vi "SpinnyGloDebugger.vi"() -> ()   [LabVIEW 2014]
uses:
  <vilib>/userdefined/High Color/IMAQdx.ctl
  <vilib>/LabVIEW Interface for Arduino/LabVIEW Interface for Arduino.lvlib
  <vilib>/vision/driver/NI_Vision_Acquisition_Software.lvlib
panel:
  in  "Camera 2 Name":T1
  out "Image 2":T2(plugin-control)
  out "Steps per Image":dbl
  out "Total Steps":dbl
  out "Images Acquired":i32
  in  "File Name":string
  in  "Save Location":path
  out "Image":T2(plugin-control)
  out "Degrees per Step":dbl
  out "Degrees per Image":dbl
  in  "Number of Images":dbl
  in  "Camera 1 Name":T1
  out "Steps Remaining":u32
  in  "Angular Increment":dbl
  in  "Exit":bool
  in  "Home":bool
  in  "Stop":bool
  in  "MoveToGo":bool
  in  "MoveForGo":bool
  in  "Direction":bool
  out "Current Position":dbl format="%#.2f"
  in  "Move For (+/-360 max)":dbl
  in  "Move To":dbl
  # "CW"
  # "CCW"
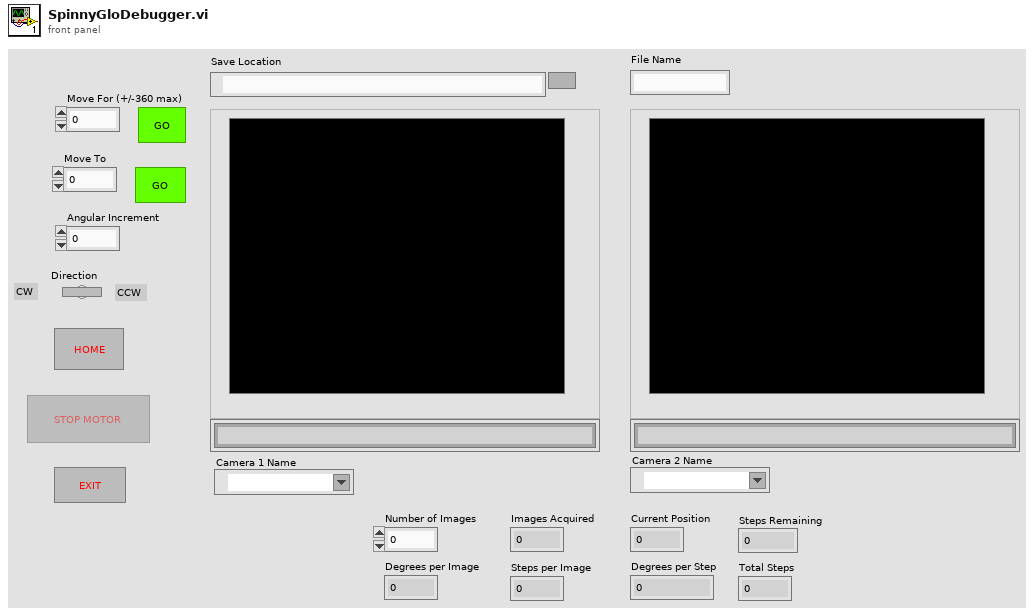
[diagram p1: front panel]
types:
  T1 = typedef "IMAQdx.ctl" = refnum<k21>
  T2 = typedef "IMAQ Image.ctl" = refnum<image>
  T3 = enum16{"Enabled", "Disabled", "Disabled and Grayed Out"}
  T4 = enum8{"Enabled", "Disabled", "Disabled and Grayed Out"}
  T5 = typedef "LabVIEW Interface for Arduino.lvlib/Arduino Resource.ctl" = cluster{"VISA resource":refnum<visa-resource-name>, "Board Type":T6, "Connection Type":enum8{"USB / Serial"}, "Bytes Per Packet (15)":u8}
  T6 = typedef "LabVIEW Interface for Arduino.lvlib/Board Type.ctl" = enum16{"Uno", "Dimuelanove w/Atmega 328", "Mega 2560"}
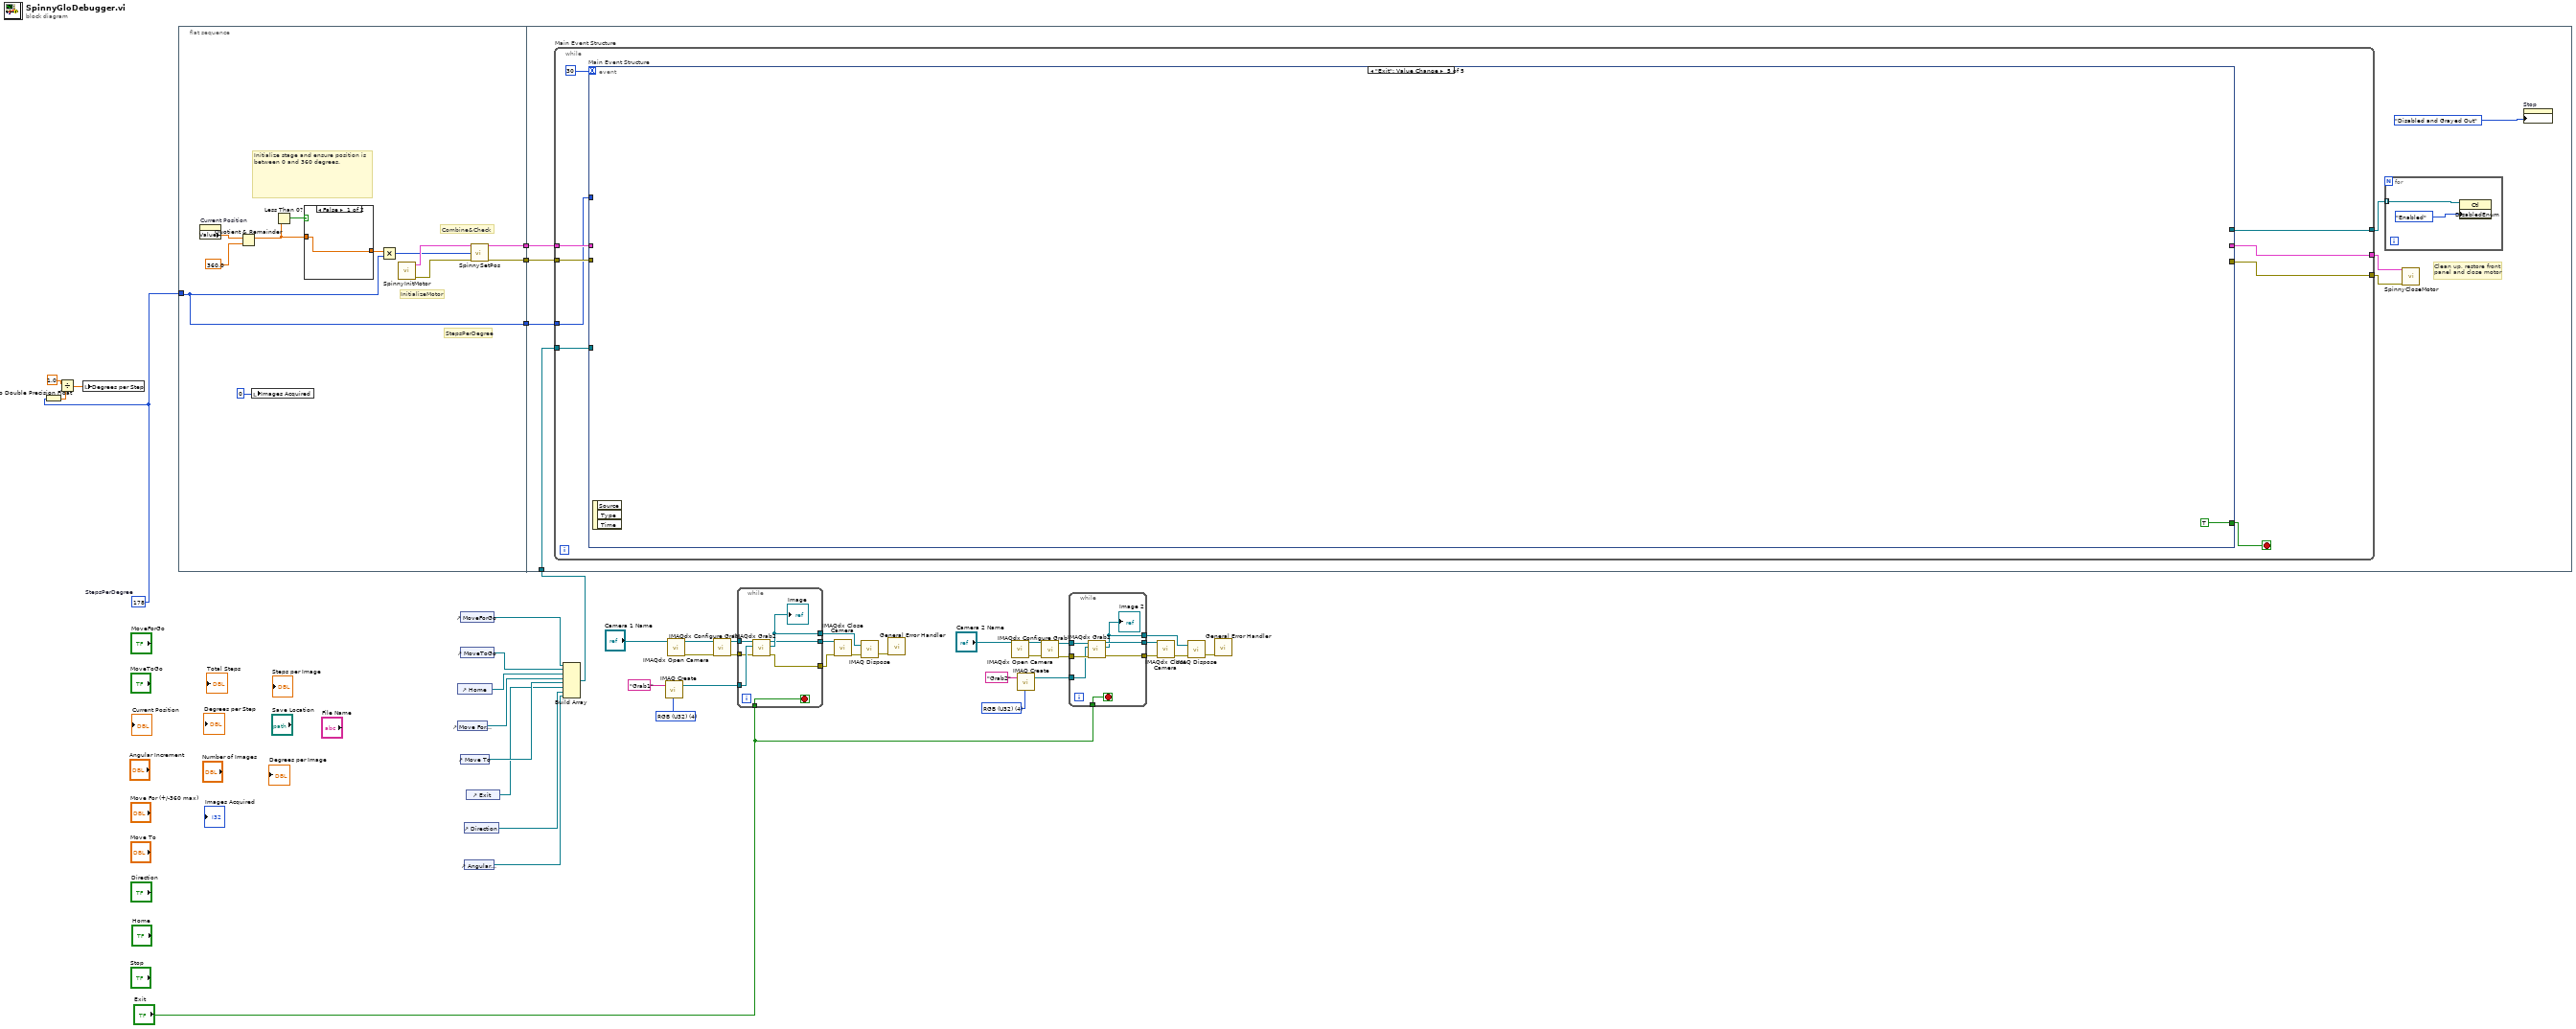
[diagram p0: block diagram]
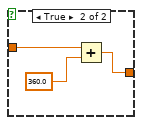
[diagram p2: hidden frame]
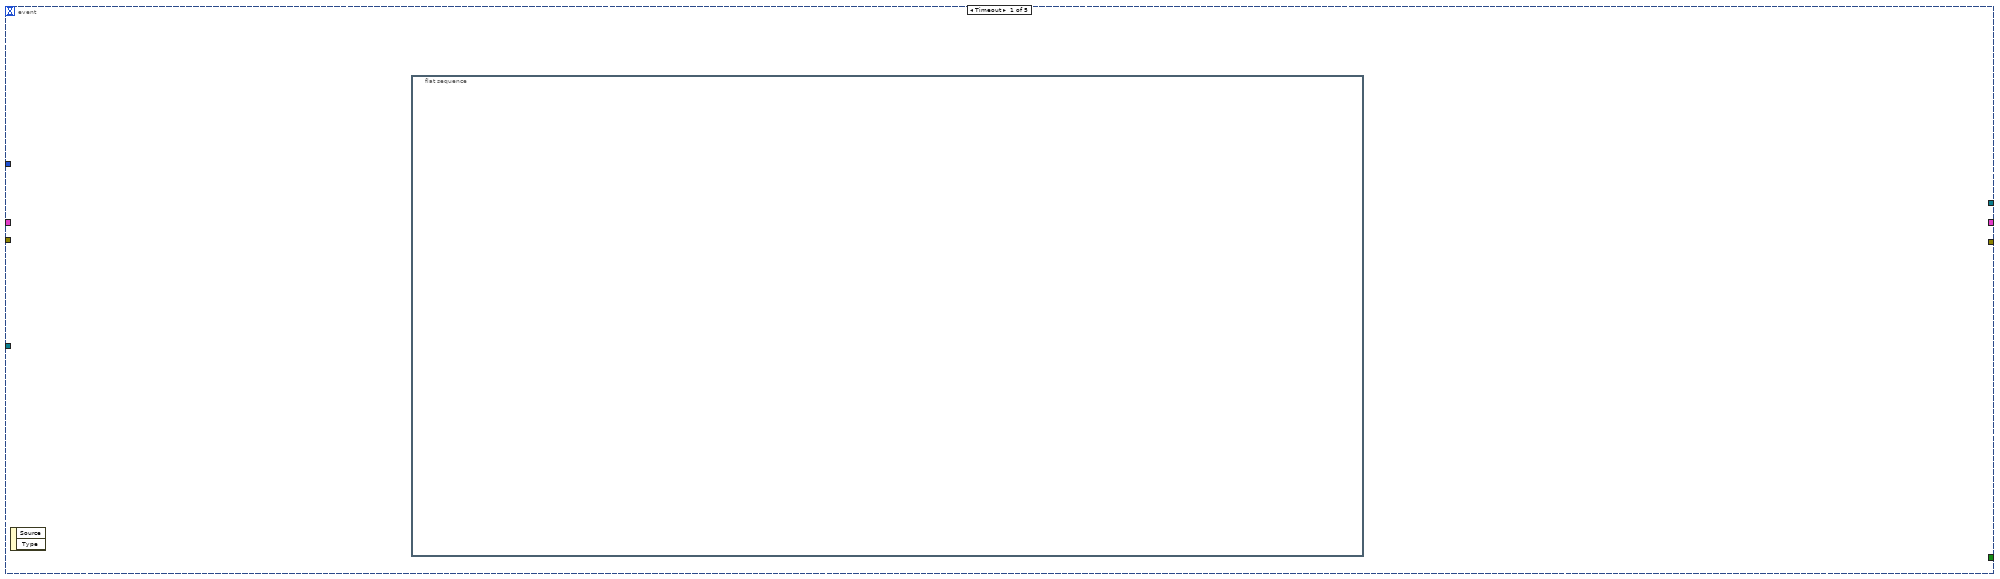
[diagram p3: hidden frame]
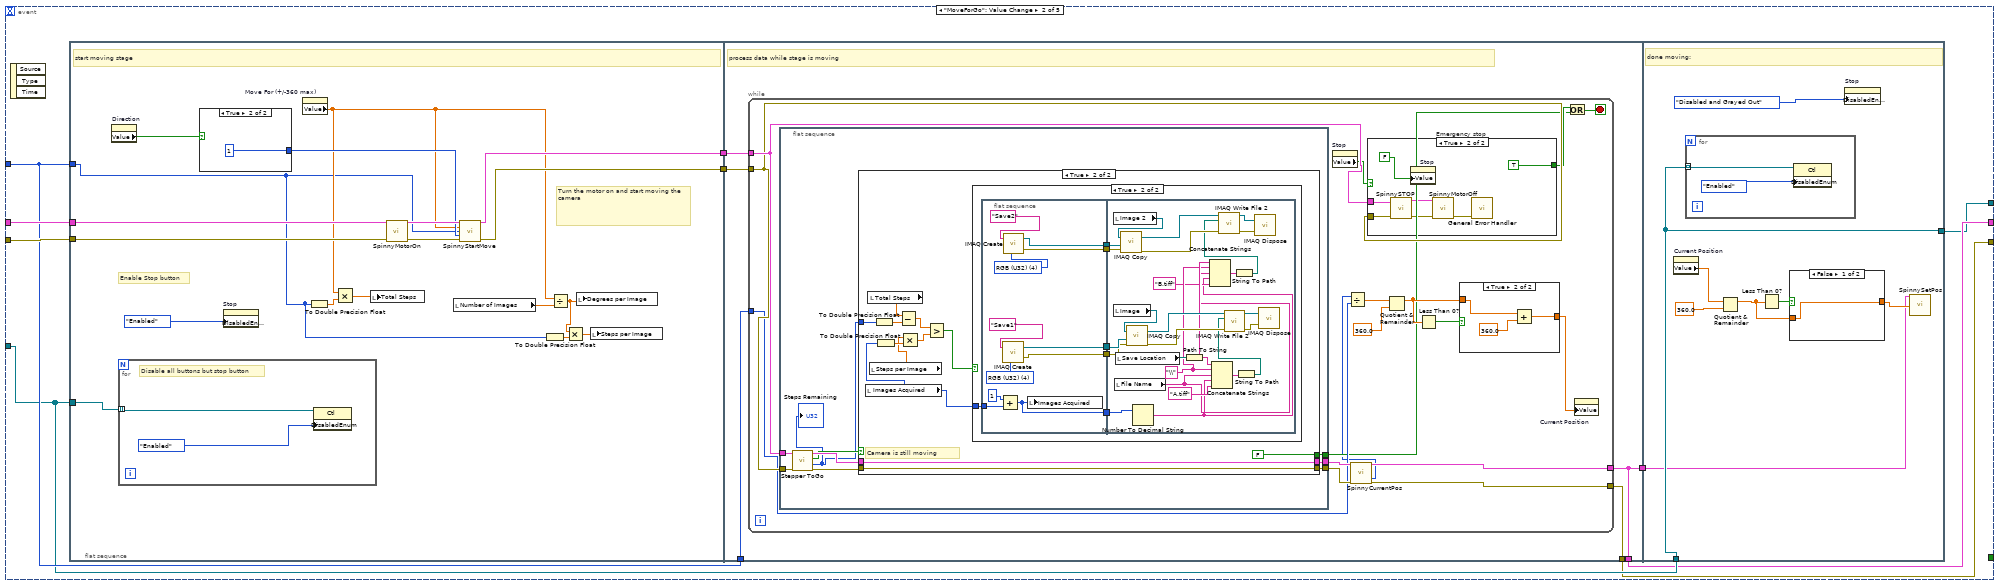
[diagram p4: hidden frame]
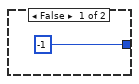
[diagram p5: hidden frame]
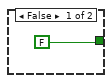
[diagram p7: hidden frame]
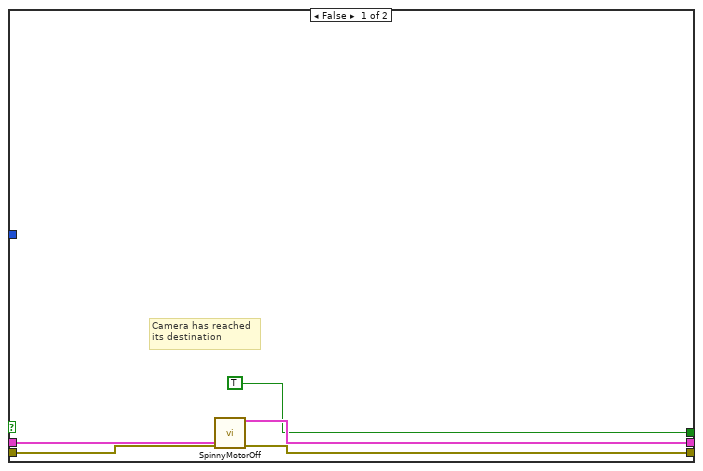
[diagram p8: hidden frame]
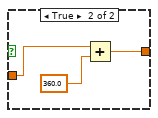
[diagram p10: hidden frame]
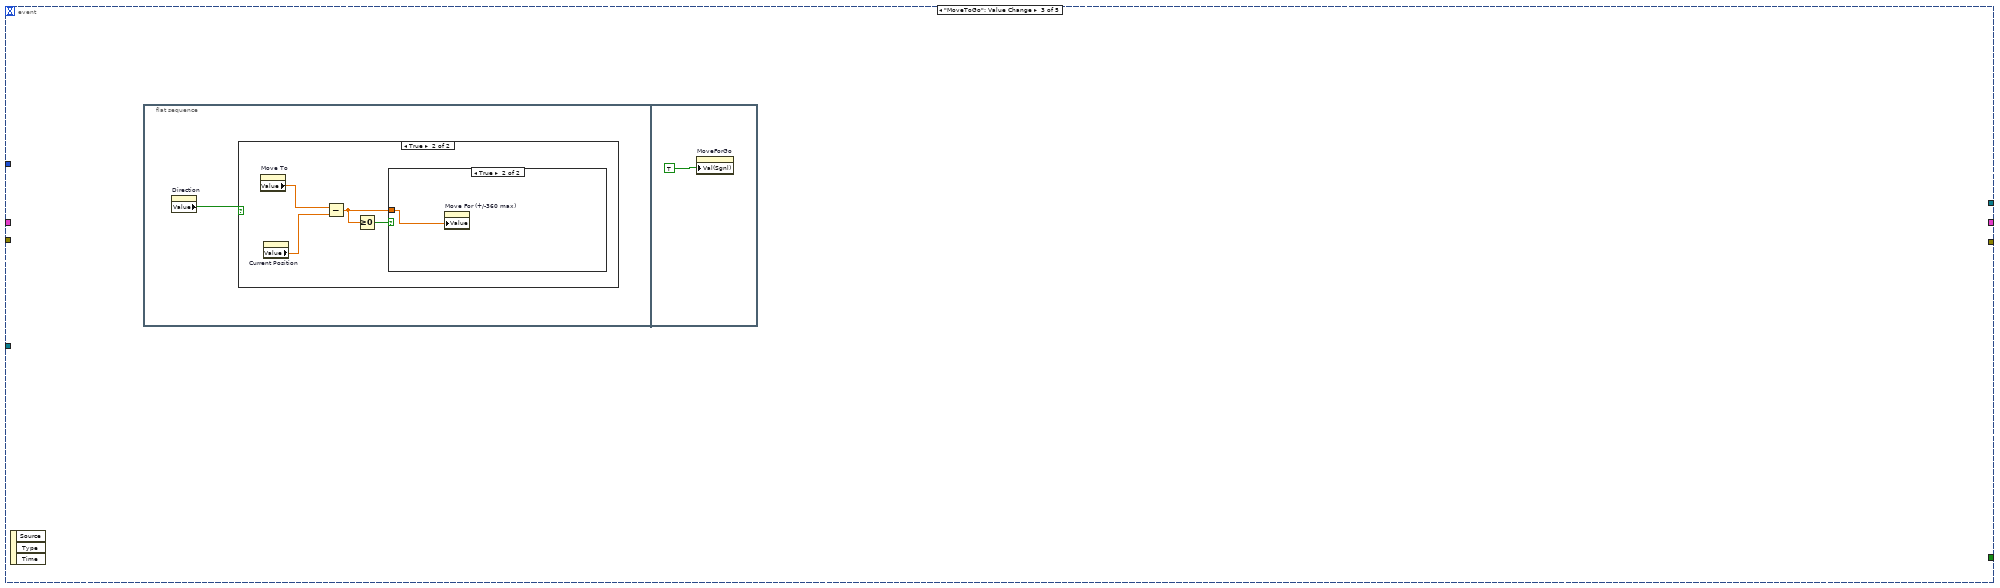
[diagram p11: hidden frame]
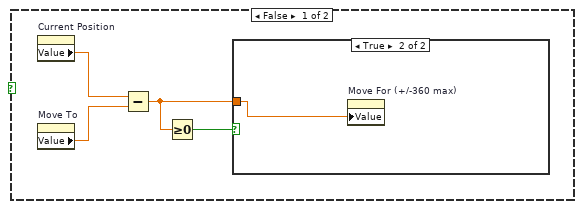
[diagram p12: hidden frame]
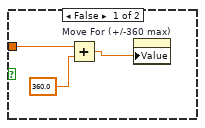
[diagram p13: hidden frame]
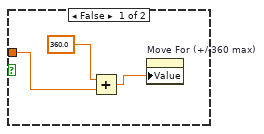
[diagram p14: hidden frame]
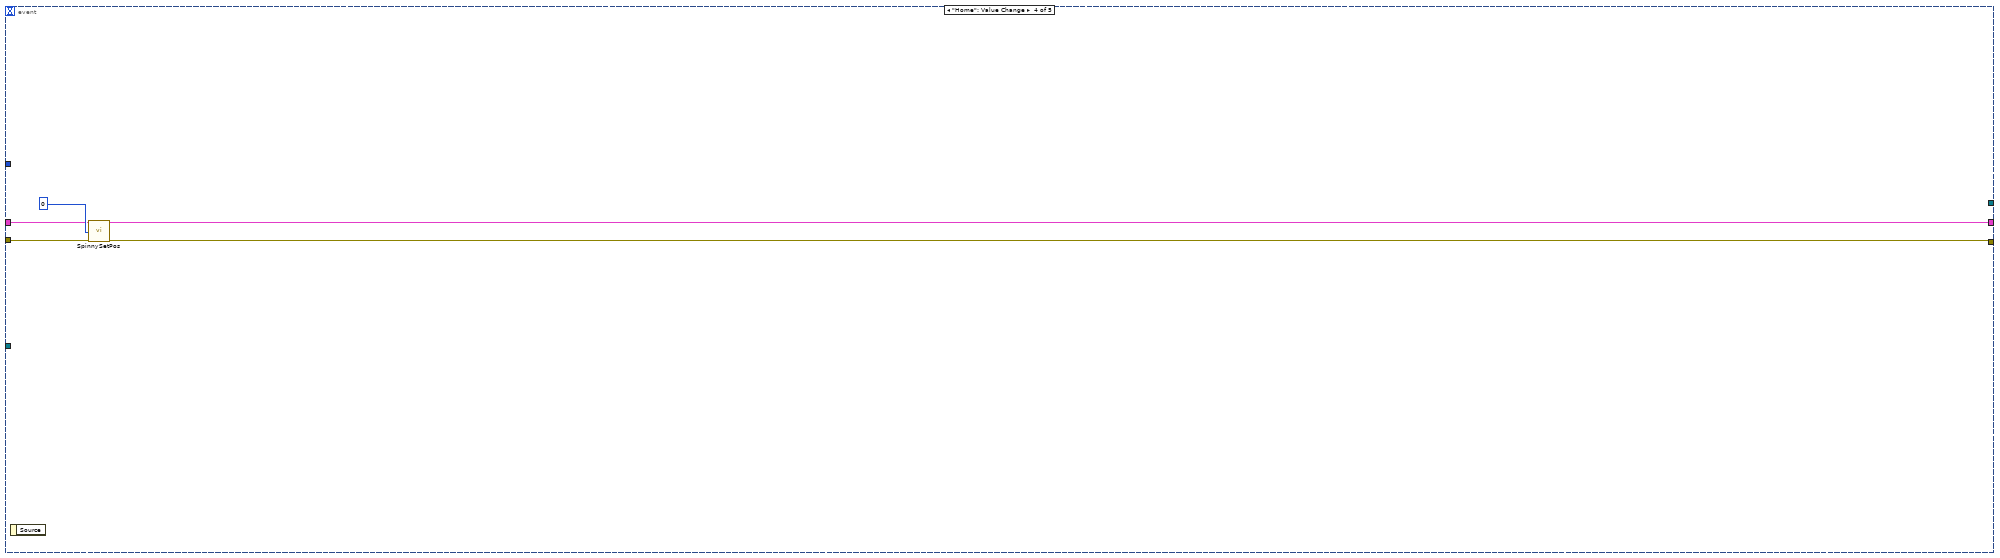
[diagram p15: hidden frame]
diagram:
  w11 = u32 4 items=["Grayscale (U8)", "Grayscale (I16)", "Grayscale (SGL)", "Complex (CSG)", "RGB (U32)", "HSL (U32)", "RGB (U64)", "Grayscale (U16)", ""] ("Image Type")
  w31 = u32 4 items=["Grayscale (U8)", "Grayscale (I16)", "Grayscale (SGL)", "Complex (CSG)", "RGB (U32)", "HSL (U32)", "RGB (U64)", "Grayscale (U16)", ""] ("Image Type")
  w15 = 178  # StepsPerDegree
  n1 = To Double Precision Float(number=w15) -> (double precision float=w18:dbl)
  n2 = Divide(x=1.0, y=w18) -> (x/y=w16:dbl)
  n3 = local write "Degrees per Step"(w16) -> ()
  n4 = flat-sequence {
    tunnel: w15 -> [w45]
    tunnel: [w47] -> w43
    tunnel: [w46] -> w42
    tunnel: [w45] -> w32
    tunnel: w43 -> [w66]
    tunnel: w42 -> [w65]
    tunnel: w33 -> [w67]
    tunnel: w32 -> [w64]
    frame #0 {
      # "StepsPerDegree"
      # "Combine&Check"
      # "InitializeMotor"
      # "Initialize stage and ensure position is between 0 and 360 degrees."
      n5 = property on="Current Position" class="DigNum (strict)"() -> ("Value"=w55:dbl)  [unwired: 2 in, 2 out]
      n6 = Quotient & Remainder(x=w55, y=sgl 360.0) -> (x-y*floor(x/y)=w52:dbl)  [unwired: 1 out]
      n7 = local write "Images Acquired"(0) -> ()
      n8 = Less Than 0?(x=w52) -> (x < 0?=w53:bool)
      n9 = case shown="False" w53 {
        tunnel: w52 -> [w56 w59]
        tunnel: [w56 w57] -> w51
        frame False {
        }
        frame True {
          n10 = Add(x=w59, y=sgl 360.0) -> (x+y=w57:dbl)
        }
      }
      n11 = Multiply(x=w51, y=w45) -> (x*y=w48:i32)
      n12 = call "SpinnyInitMotor.vi"() -> ("error out"=w49:errorcluster, "Arduino Resource Out"=w50:T5)  [unwired: 10 in]
      n13 = call "SpinnySetPos.vi"("Arduino Resource"=w50, "position"=w48, "error in"=w49) -> ("Arduino Resource Out"=w47:T5, "error out"=w46:errorcluster)  [unwired: 15 in]
    }
    frame #1 {
      # "Clean up, restore front\npanel and close motor"
      n14 = while "Main Event Structure" {
        tunnel: w67 -> [w77]
        tunnel: w66 -> [w76]
        tunnel: w65 -> [w75]
        tunnel: w64 -> [w74]
        tunnel: [w73] -> w61
        tunnel: [w72] -> w63
        tunnel: [w71] -> w62
        stop <- w70 stop-if-true
        n15 = event "Main Event Structure" shown="[4] \"Exit\": Value Change" {
          selector: _ -> [_ _ _ _ _]
          dyn-events: _ -> [_ _ _ _ _]
          timeout: 30 -> [_ _ _ _ _]
          tunnel: w77 -> [_ w82 _ _ _]
          tunnel: w76 -> [_ w88 _ w249 _]
          tunnel: w75 -> [_ w87 _ w248 _]
          tunnel: w74 -> [_ w84 _ _ _]
          tunnel: [_ w81 _ w247 _] -> w72
          tunnel: [_ w80 _ w246 _] -> w71
          tunnel: [_ w79 _ _ _] -> w73
          tunnel: [_ _ _ _ TRUE] -> w70
          event Timeout {
            n16 = event-data() -> ()  [unwired: 1 in, 2 out]
            n17 = flat-sequence {
              frame #0 {
              }
            }
          }
          event "MoveForGo": Value Change {
            n18 = event-data() -> ()  [unwired: 1 in, 3 out]
            n19 = flat-sequence {
              tunnel: w82 -> [w106]
              tunnel: w88 -> [w103]
              tunnel: w87 -> [w101]
              tunnel: w84 -> [w92]
              tunnel: [w98] -> w86
              tunnel: [w97] -> w85
              tunnel: w86 -> [w115]
              tunnel: w85 -> [w114]
              tunnel: w84 -> [w113]
              tunnel: [w112] -> w83
              tunnel: [w112] -> w81
              tunnel: [w111] -> w80
              tunnel: w83 -> [w214]
              tunnel: w82 -> [w215]
              tunnel: [w215] -> w79
              frame #0 {
                # "Turn the motor on and start moving the camera"
                # "start moving stage"
                # "Enable Stop button"
                n20 = property on="Direction" class="Bool (strict)"() -> ("Value"=w104:bool)  [unwired: 2 in, 2 out]
                n21 = for {
                  tunnel: w106 -> [w110] mode=indexing
                  # "Disable all buttons but stop button"
                  n22 = property class="Ctl"(reference=w110, "DisabledEnum"=T3."Enabled") -> ()  [unwired: 1 in, 2 out]
                }
                n23 = case shown="True" w104 {
                  tunnel: [-1 1] -> w99
                  frame False {
                  }
                  frame True {
                  }
                }
                n24 = property on="Stop" class="Bool (strict)"("DisabledEnum"=T4."Enabled") -> ()  [unwired: 2 in, 2 out]
                n25 = property on="Move For (+/-360 max)" class="DigNum (strict)"() -> ("Value"=w94:dbl)  [unwired: 2 in, 2 out]
                n26 = To Double Precision Float(number=w92) -> (double precision float=w95:dbl)
                n27 = Multiply(x=w94, y=w95) -> (x*y=w93:dbl)
                n28 = local write "Total Steps"(w93) -> ()
                n29 = call "SpinnyMotorOn.vi"("Arduino Resource"=w103, "error in"=w101) -> ("Arduino Resource Out"=w102:T5, "error out"=w100:errorcluster)  [unwired: 12 in]
                n30 = local read "Number of Images"() -> (w96:dbl)
                n31 = call "SpinnyStartMove.vi"("Arduino Resource"=w102, "Degrees To Move"=w94, "Steps Per Degree"=w92, "Direction"=w99, "error in"=w100) -> ("Arduino Resource Out"=w98:T5, "error out"=w97:errorcluster)  [unwired: 9 in]
                n32 = To Double Precision Float(number=w92) -> (double precision float=w91:dbl)
                n33 = Divide(x=w94, y=w96) -> (x/y=w90:dbl)
                n34 = Multiply(x=w90, y=w91) -> (x*y=w89:dbl)
                n35 = local write "Degrees per Image"(w90) -> ()
                n36 = local write "Steps per Image"(w89) -> ()
              }
              frame #1 {
                # "process data while stage is moving"
                n37 = while {
                  tunnel: w115 -> [w130]
                  tunnel: w114 -> [w129]
                  tunnel: [w128] -> w111
                  tunnel: [w126] -> w112
                  tunnel: w113 -> [w125]
                  stop <- w118 stop-if-true
                  n38 = flat-sequence {
                    tunnel: w129 -> [w153]
                    tunnel: w130 -> [w152]
                    tunnel: [w148] -> w131
                    tunnel: [w147] -> w132
                    tunnel: [w146] -> w119
                    frame #0 {
                      n39 = call <vilib>:"Stepper ToGo.vi"("error in"=w153, "Arduino Resource"=w152) -> ("error out"=w150:errorcluster, "Steps remaining"=w145:u32, "Steps Remaining?"=w149:bool, "Arduino Resource Out"=w151:T5)  [unwired: 6 in]
                      "Steps Remaining" <- w145
                      n40 = case shown="True" w149 {
                        tunnel: w151 -> [w158 w170]
                        tunnel: w150 -> [w157 w169]
                        tunnel: [w156 w170] -> w147
                        tunnel: [w155 w169] -> w148
                        tunnel: [TRUE FALSE] -> w146
                        tunnel: w145 -> [_ w167]
                        frame False {
                          # "Camera has reached\nits destination"
                          n41 = call "SpinnyMotorOff.vi"("Arduino Resource"=w158, "error in"=w157) -> ("Arduino Resource Out"=w156:T5, "error out"=w155:errorcluster)  [unwired: 12 in]
                        }
                        frame True {
                          # "Camera is still moving"
                          n42 = local read "Images Acquired"() -> (w161:i32)
                          n43 = local read "Total Steps"() -> (w165:dbl)
                          n44 = local read "Steps per Image"() -> (w160:dbl)
                          n45 = To Double Precision Float(number=w167) -> (double precision float=w166:dbl)
                          n46 = To Double Precision Float(number=w161) -> (double precision float=w162:dbl)
                          n47 = Subtract(x=w165, y=w166) -> (x-y=w164:dbl)
                          n48 = Multiply(x=w160, y=w162) -> (x*y=w159:dbl)
                          n49 = Greater?(x=w164, y=w159) -> (0:w163:bool)
                          n50 = case shown="True" w163 {
                            tunnel: w161 -> [_ w174]
                            frame False {
                            }
                            frame True {
                              n51 = flat-sequence {
                                tunnel: [w185] -> w176
                                tunnel: [w184] -> w175
                                tunnel: w174 -> [w183]
                                tunnel: [w181] -> w173
                                tunnel: [w178] -> w172
                                tunnel: [w177] -> w171
                                tunnel: w176 -> [w212]
                                tunnel: w175 -> [w208]
                                tunnel: w173 -> [w204]
                                tunnel: w172 -> [w195]
                                tunnel: w171 -> [w194]
                                frame #0 {
                                w179 = u16 4 items=["Grayscale (U8)", "Grayscale (I16)", "Grayscale (SGL)", "Complex (CSG)", "RGB (U32)", "HSL (U32)", "RGB (U64)", "Grayscale (U16)", ""]
                                w186 = u16 4 items=["Grayscale (U8)", "Grayscale (I16)", "Grayscale (SGL)", "Complex (CSG)", "RGB (U32)", "HSL (U32)", "RGB (U64)", "Grayscale (U16)", ""]
                                n52 = Add(x=1, y=w183) -> (x+y=w181:i32)
                                n53 = call "IMAQ Create"("Image Name"="Save1", "Image Type"=w186) -> ("New Image"=w185:T2, "error out"=w184:errorcluster)  [unwired: 3 in]
                                n54 = call "IMAQ Create"("Image Name"="Save2", "Image Type"=w179) -> ("New Image"=w178:T2, "error out"=w177:errorcluster)  [unwired: 3 in]
                                n55 = local write "Images Acquired"(w181) -> ()
                                }
                                frame #1 {
                                w200 = "\\"
                                n56 = local read "Image 2"() -> (w196:T2)
                                n57 = local read "Image"() -> (w213:T2)
                                n58 = local read "File Name"() -> (w199:string)
                                n59 = local read "Save Location"() -> (w206:path)
                                n60 = call "IMAQ Copy"("error in (no error)"=w194, "Image Dst"=w195, "Image Src"=w196) -> ("error out"=w193:errorcluster, "Image Dst Out"=w191:T2)  [unwired: 3 in]
                                n61 = call "IMAQ Copy"("error in (no error)"=w208, "Image Dst"=w212, "Image Src"=w213) -> ("error out"=w207:errorcluster, "Image Dst Out"=w211:T2)  [unwired: 3 in]
                                n62 = Number To Decimal String(number=w204) -> (decimal integer string=w197:string)  [unwired: 1 in]
                                n63 = Path To String(path=w206) -> (string=w201:string)
                                n64 = Concatenate Strings(w201, w200, w199, w197, "B.tiff") -> (w189:string)
                                n65 = Concatenate Strings(w201, w200, w199, w197, "A.tiff") -> (w203:string)
                                n66 = String To Path(string=w189) -> (path=w188:path)
                                n67 = call-poly "IMAQ Write File 2"("error in (no error)"=w193, "File Path"=w188, "Image"=w191) -> ("error out"=w192:errorcluster, "Image Out (duplicate)"=w190:T2)  [unwired: 7 in]
                                n68 = String To Path(string=w203) -> (path=w202:path)
                                n69 = call-poly "IMAQ Write File 2"("error in (no error)"=w207, "File Path"=w202, "Image"=w211) -> ("error out"=w209:errorcluster, "Image Out (duplicate)"=w210:T2)  [unwired: 7 in]
                                n70 = call "IMAQ Dispose"("Image"=w190, "error in (no error)"=w192) -> ()  [unwired: 4 in, 1 out]
                                n71 = call "IMAQ Dispose"("Image"=w210, "error in (no error)"=w209) -> ()  [unwired: 4 in, 1 out]
                                }
                              }
                            }
                          }
                        }
                      }
                    }
                  }
                  n72 = property on="Stop" class="Bool (strict)"() -> ("Value"=w127:bool)  [unwired: 2 in, 2 out]
                  n73 = call "SpinnyCurrentPos.vi"("Arduino Resource"=w132, "error in"=w131) -> ("Arduino Resource Out"=w126:T5, "position"=w116:i32, "error out"=w128:errorcluster)  [unwired: 15 in]
                  n74 = Divide(x=w116, y=w125) -> (x/y=w124:dbl)
                  n75 = case "Emergency stop" shown="True" w127 {
                    tunnel: w130 -> [_ w144]
                    tunnel: w129 -> [_ w142]
                    tunnel: [FALSE TRUE] -> w120
                    frame False {
                    }
                    frame True {
                      n76 = call "SpinnySTOP.vi"("error in"=w142, "Arduino Resource"=w144) -> ("error out"=w141:errorcluster, "Arduino Resource Out"=w143:T5)  [unwired: 8 in]
                      n77 = property on="Stop" class="Bool (strict)"("Value"=FALSE) -> ()  [unwired: 2 in, 2 out]
                      n78 = call "SpinnyMotorOff.vi"("Arduino Resource"=w143, "error in"=w141) -> ("error out"=w140:errorcluster)  [unwired: 12 in, 1 out]
                      n79 = call <vilib>:"General Error Handler.vi"("error in (no error)"=w140) -> ()  [unwired: 10 in, 5 out]
                    }
                  }
                  n80 = Quotient & Remainder(x=w124, y=sgl 360.0) -> (x-y*floor(x/y)=w122:dbl)  [unwired: 1 out]
                  n81 = Less Than 0?(x=w122) -> (x < 0?=w121:bool)
                  n82 = case shown="True" w121 {
                    tunnel: w122 -> [w133 w135]
                    tunnel: [w133 w134] -> w117
                    frame False {
                    }
                    frame True {
                      n83 = Add(x=w135, y=sgl 360.0) -> (x+y=w134:dbl)
                    }
                  }
                  n84 = Or(x=w120, y=w119) -> (x .or. y?=w118:bool)
                  n85 = property on="Current Position" class="DigNum (strict)"("Value"=w117) -> ()  [unwired: 2 in, 2 out]
                }
              }
              frame #2 {
                # "done moving:"
                n86 = property on="Current Position" class="DigNum (strict)"() -> ("Value"=w220:dbl)  [unwired: 2 in, 2 out]
                n87 = for {
                  tunnel: w215 -> [w226] mode=indexing
                  n88 = property class="Ctl"(reference=w226, "DisabledEnum"=T3."Enabled") -> ()  [unwired: 1 in, 2 out]
                }
                n89 = Quotient & Remainder(x=w220, y=sgl 360.0) -> (x-y*floor(x/y)=w217:dbl)  [unwired: 1 out]
                n90 = Less Than 0?(x=w217) -> (x < 0?=w218:bool)
                n91 = case shown="False" w218 {
                  tunnel: w217 -> [w222 w225]
                  tunnel: [w222 w223] -> w216
                  frame False {
                  }
                  frame True {
                    n92 = Add(x=w225, y=sgl 360.0) -> (x+y=w223:dbl)
                  }
                }
                n93 = property on="Stop" class="Bool (strict)"("DisabledEnum"=T3."Disabled and Grayed Out") -> ()  [unwired: 2 in, 2 out]
                n94 = call "SpinnySetPos.vi"("Arduino Resource"=w214, "position"=w216) -> ()  [unwired: 16 in, 2 out]
              }
            }
          }
          event "MoveToGo": Value Change {
            n95 = event-data() -> ()  [unwired: 1 in, 3 out]
            n96 = flat-sequence {
              frame #0 {
                n97 = property on="Direction" class="Bool (strict)"() -> ("Value"=w228:bool)  [unwired: 2 in, 2 out]
                n98 = case shown="True" w228 {
                  frame False {
                    n99 = property on="Current Position" class="DigNum (strict)"() -> ("Value"=w231:dbl)  [unwired: 2 in, 2 out]
                    n100 = property on="Move To" class="DigNum (strict)"() -> ("Value"=w232:dbl)  [unwired: 2 in, 2 out]
                    n101 = Subtract(x=w231, y=w232) -> (x-y=w229:dbl)
                    n102 = Greater Or Equal To 0?(x=w229) -> (x >= 0?=w230:bool)
                    n103 = case shown="True" w230 {
                      tunnel: w229 -> [w234 w236]
                      frame False {
                        n104 = Add(x=w234, y=sgl 360.0) -> (x+y=w233:dbl)
                        n105 = property on="Move For (+/-360 max)" class="DigNum (strict)"("Value"=w233) -> ()  [unwired: 2 in, 2 out]
                      }
                      frame True {
                        n106 = property on="Move For (+/-360 max)" class="DigNum (strict)"("Value"=w236) -> ()  [unwired: 2 in, 2 out]
                      }
                    }
                  }
                  frame True {
                    n107 = property on="Move To" class="DigNum (strict)"() -> ("Value"=w239:dbl)  [unwired: 2 in, 2 out]
                    n108 = property on="Current Position" class="DigNum (strict)"() -> ("Value"=w240:dbl)  [unwired: 2 in, 2 out]
                    n109 = Subtract(x=w239, y=w240) -> (x-y=w238:dbl)
                    n110 = Greater Or Equal To 0?(x=w238) -> (x >= 0?=w237:bool)
                    n111 = case shown="True" w237 {
                      tunnel: w238 -> [w242 w244]
                      frame False {
                        n112 = Add(x=sgl 360.0, y=w242) -> (x+y=w243:dbl)
                        n113 = property on="Move For (+/-360 max)" class="DigNum (strict)"("Value"=w243) -> ()  [unwired: 2 in, 2 out]
                      }
                      frame True {
                        n114 = property on="Move For (+/-360 max)" class="DigNum (strict)"("Value"=w244) -> ()  [unwired: 2 in, 2 out]
                      }
                    }
                  }
                }
              }
              frame #1 {
                n115 = property on="MoveForGo" class="Bool (strict)"("Val(Sgnl)"=TRUE) -> ()  [unwired: 2 in, 2 out]
              }
            }
          }
          event "Home": Value Change {
            n116 = event-data() -> ()  [unwired: 1 in, 1 out]
            n117 = call "SpinnySetPos.vi"("Arduino Resource"=w249, "position"=0, "error in"=w248) -> ("Arduino Resource Out"=w247:T5, "error out"=w246:errorcluster)  [unwired: 15 in]
          }
          event "Exit": Value Change {
            n118 = event-data() -> ()  [unwired: 1 in, 3 out]
          }
        }
      }
      n119 = for {
        tunnel: w61 -> [w68] mode=indexing
        n120 = property class="Ctl"(reference=w68, "DisabledEnum"=T3."Enabled") -> ()  [unwired: 1 in, 2 out]
      }
      n121 = call "SpinnyCloseMotor.vi"("Arduino Resource"=w63, "error in"=w62) -> ()  [unwired: 18 in]
      n122 = property on="Stop" class="Bool (strict)"("DisabledEnum"=T3."Disabled and Grayed Out") -> ()  [unwired: 2 in, 2 out]
    }
  }
  n123 = control-ref of="Home"() -> (w39:refnum<vi>)
  n124 = control-ref of="Move For (+/-360 max)"() -> (w38:refnum<vi>)
  n125 = control-ref of="MoveForGo"() -> (w41:refnum<vi>)
  n126 = control-ref of="MoveToGo"() -> (w40:refnum<vi>)
  n127 = control-ref of="Move To"() -> (w37:refnum<vi>)
  n128 = control-ref of="Direction"() -> (w35:refnum<vi>)
  n129 = control-ref of="Angular Increment"() -> (w34:refnum<vi>)
  n130 = control-ref of="Exit"() -> (w36:refnum<vi>)
  n131 = Build Array(w41, w40, w39, w38, w37, w36, w35, w34) -> (w33:refnum<vi>[])
  n132 = call "IMAQ Create"("Image Name"="Grab1", "Image Type"=w31) -> ("New Image"=w25:T2)  [unwired: 3 in, 1 out]
  n133 = call <vilib>:"IMAQdx Open Camera.vi"("Session In"="Camera 1 Name") -> ("error out"=w28:errorcluster, "Session Out"=w27:T1)  [unwired: 9 in]
  n134 = call <vilib>:"IMAQdx Configure Grab.vi"("error in"=w28, "Session In"=w27) -> ("error out"=w24:errorcluster, "Session Out"=w26:T1)  [unwired: 8 in]
  n135 = while {
    tunnel: w26 -> [w258]
    tunnel: w25 -> [w257]
    tunnel: w24 -> [w256]
    tunnel: [w255] -> w23
    tunnel: [w254] -> w20
    tunnel: [w253] -> w19
    tunnel: "Exit" -> [w252]
    stop <- w252 stop-if-true
    n136 = call <vilib>:"IMAQdx Grab2.vi"("error in"=w256, "Image In"=w257, "Session In"=w258) -> ("error out"=w255:errorcluster, "Image Out"=w254:T2, "Session Out"=w253:T1)  [unwired: 5 in, 1 out]
    "Image" <- w254
  }
  n137 = call <vilib>:"IMAQdx Close Camera.vi"("error in"=w23, "Session In"=w19) -> ("error out"=w22:errorcluster)  [unwired: 9 in]
  n138 = call "IMAQ Dispose"("Image"=w20, "error in (no error)"=w22) -> ("error out"=w21:errorcluster)  [unwired: 4 in]
  n139 = call <vilib>:"General Error Handler.vi"("error in (no error)"=w21) -> ()  [unwired: 10 in, 5 out]
  n140 = call <vilib>:"IMAQdx Open Camera.vi"("Session In"="Camera 2 Name") -> ("error out"=w12:errorcluster, "Session Out"=w13:T1)  [unwired: 9 in]
  n141 = call "IMAQ Create"("Image Name"="Grab2", "Image Type"=w11) -> ("New Image"=w7:T2)  [unwired: 3 in, 1 out]
  n142 = call <vilib>:"IMAQdx Configure Grab.vi"("error in"=w12, "Session In"=w13) -> ("error out"=w8:errorcluster, "Session Out"=w9:T1)  [unwired: 8 in]
  n143 = while {
    tunnel: w9 -> [w265]
    tunnel: w8 -> [w264]
    tunnel: w7 -> [w263]
    tunnel: [w262] -> w6
    tunnel: [w261] -> w3
    tunnel: [w260] -> w2
    tunnel: "Exit" -> [w259]
    stop <- w259 stop-if-true
    n144 = call <vilib>:"IMAQdx Grab2.vi"("error in"=w264, "Image In"=w263, "Session In"=w265) -> ("error out"=w262:errorcluster, "Image Out"=w260:T2, "Session Out"=w261:T1)  [unwired: 5 in, 1 out]
    "Image 2" <- w260
  }
  n145 = call <vilib>:"IMAQdx Close Camera.vi"("error in"=w6, "Session In"=w3) -> ("error out"=w5:errorcluster)  [unwired: 9 in]
  n146 = call "IMAQ Dispose"("Image"=w2, "error in (no error)"=w5) -> ("error out"=w4:errorcluster)  [unwired: 4 in]
  n147 = call <vilib>:"General Error Handler.vi"("error in (no error)"=w4) -> ()  [unwired: 10 in, 5 out]
